vi "Suite from Test Case Path.vi"(7 "Ignore Index?":bool, 8 "error in (no error)":errorcluster, 10 "Test Case":path) -> (0 "error out":errorcluster, 3 "LUnit Test Suite Out":refnum<class "LUnit Test Suite.lvclass">)   [LabVIEW 2020, in "Test Finder.lvclass"]
doc: "Produce a test suite including all test methods in a single test case class."
uses:
  Test Finder.lvclass
  LUnit Test Suite.lvclass
  LUnit Test Case.lvclass
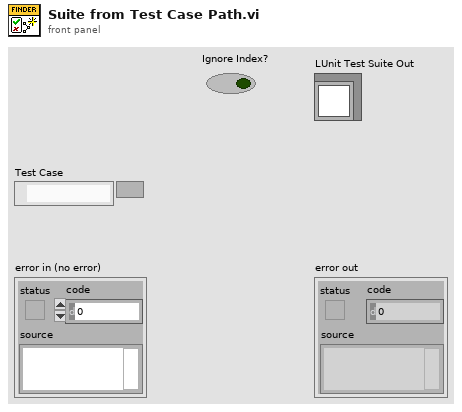
[diagram p1: front panel]
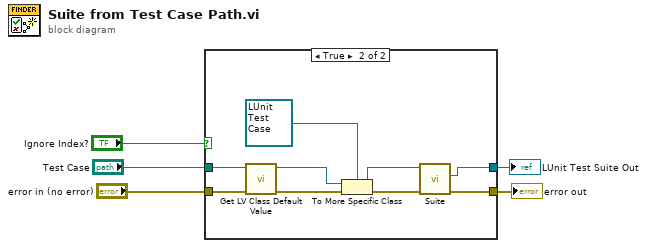
[diagram p0: block diagram]
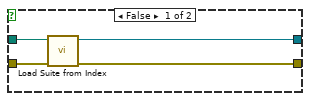
[diagram p2: hidden frame]
diagram:
  n1 = case shown="True" "Ignore Index?" {
    tunnel: [w9 w17] -> w5
    tunnel: [w8 w16] -> w4
    tunnel: "Test Case" -> [w7 w15]
    tunnel: "error in (no error)" -> [w6 w18]
    frame False {
      n2 = call "Load Suite from Index.vi"("error in (no error)"=w6, "Path"=w7) -> ("error out"=w9:errorcluster, "LUnit Test Suite out"=w8:refnum<class "LUnit Test Suite.lvclass">)  [unwired: 8 in]
    }
    frame True {
      n3 = call <vilib>:"Get LV Class Default Value.vi"("error in (no error)"=w18, "class path"=w15) -> ("error out"=w12:errorcluster, "object"=w11:refnum<class>)  [unwired: 8 in]
      n4 = To More Specific Class(target class=refnum<class "LUnit Test Case.lvclass"> refnum ("LUnit Test Case.lvclass"), reference=w11, error in=w12) -> (specific class reference=w14:refnum<class "LUnit Test Case.lvclass">, error out=w13:errorcluster)
      n5 = call-dynamic "Suite.vi"("error in (no error)"=w13, "LUnit Test Case In"=w14) -> ("error out"=w17:errorcluster, "LUnit Test Suite Out"=w16:refnum<class "LUnit Test Suite.lvclass">)  [unwired: 7 in, 1 out]
    }
  }
  "error out" <- w5
  "LUnit Test Suite Out" <- w4
